vi "Wait for Lifter.vi"(9 "1 tote high":dbl, 10 "Auto Lifter States":T1, 11 "MechanismMetrics in in":T2) -> (3 "MechanismMetrics out":T2)   [LabVIEW 2014]
uses:
  MechanismMetrics.ctl
  Lifter States.ctl
  Auto Lifter States.ctl
  encoderData.vi
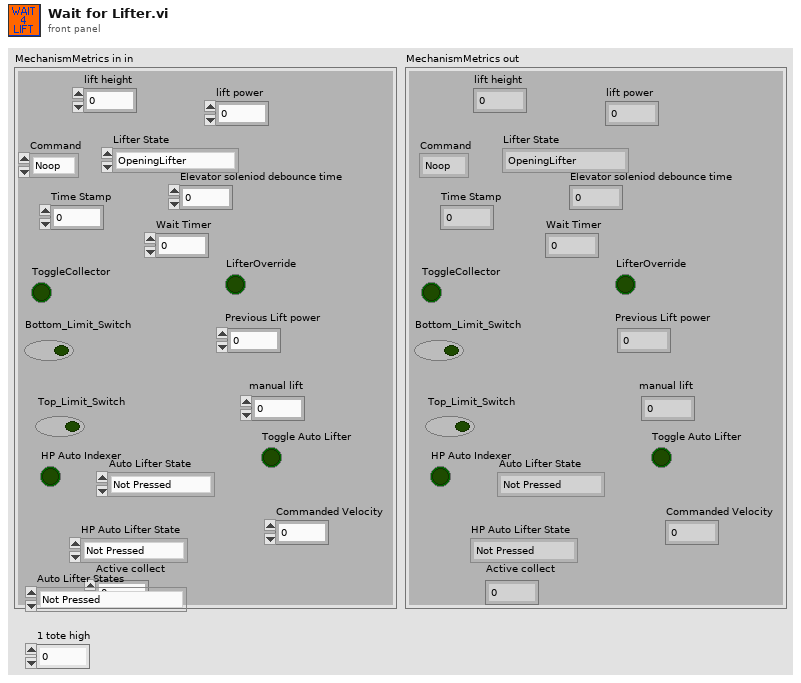
[diagram p1: front panel]
types:
  T1 = typedef "Auto Lifter States.ctl" = enum16{"Not Pressed", "THE_END", "WAIT_FOR_RELEASE", "Press Detected", "To Release Stacked1", "To Collect", "Open Lifter", "WAIT", "Close", "To Stack1"}
  T2 = typedef "MechanismMetrics.ctl" = cluster{"lift height":dbl, "Command":enum16{"Noop", "Flagged"}, "Time Stamp":u32, "ToggleCollector":bool, "Bottom_Limit_Switch ":bool, "Top_Limit_Switch":bool, "lift power":dbl, "Elevator soleniod debounce time   ":dbl, "LifterOverride":bool, "Previous Lift power":dbl, "manual lift":dbl, "Lifter State":T3, "Auto Lifter State":T1, "Toggle Auto Lifter":bool, "Wait Timer":dbl, "HP Auto Indexer":bool, "HP Auto Lifter State":T1, "Commanded Velocity":dbl, "\nActive collect":dbl}
  T3 = typedef "Lifter States.ctl" = enum16{"OpeningLifter", "LifterOpen", "ClosingLifter", "LifterClosed"}
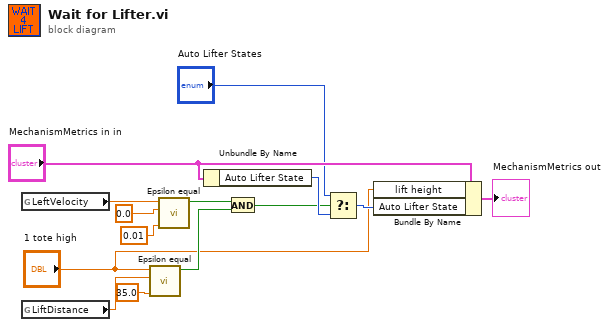
[diagram p0: block diagram]
diagram:
  n1 = global read "encoderData.vi" "LeftVelocity"() -> (w4:dbl)
  n2 = global read "encoderData.vi" "LiftDistance"() -> (w1:dbl)
  n3 = call "Epsilon equal.vi"("Epsilon"=35.0, "Value2"=w1, "Value1"="1 tote high") -> ("Boolean"=w8:bool)  [unwired: 8 in]
  n4 = call "Epsilon equal.vi"("Epsilon"=0.01, "Value2"=0.0, "Value1"=w4) -> ("Boolean"=w7:bool)  [unwired: 8 in]
  n5 = Unbundle By Name("MechanismMetrics in in") -> ("Auto Lifter State"=w12:T1)
  n6 = And(x=w7, y=w8) -> (x .and. y?=w9:bool)
  n7 = Select(t="Auto Lifter States", s=w9, f=w12) -> (s? t:f=w13:T1)
  n8 = Bundle By Name(cluster="MechanismMetrics in in", "lift height"="1 tote high", "Auto Lifter State"=w13) -> (→"MechanismMetrics out":T2)
